vi "SetNeoPixelBrightness.vi"(8 "error in (no error)":errorcluster, 10 "Brightness":u8, 11 "AdaFruit-Seesaw in":refnum<class "AdaFruit-Seesaw.lvclass">) -> (0 "error out":errorcluster, 3 "AdaFruit-Seesaw out":refnum<class "AdaFruit-Seesaw.lvclass">)   [LabVIEW 2020, in "CTI-Peripheral.lvlib" / "AdaFruit-Seesaw.lvclass"]
uses:
  AdaFruit-Seesaw.lvclass
  AdaFruit-Seesaw.lvclass/AdaFruit-Seesaw.ctl
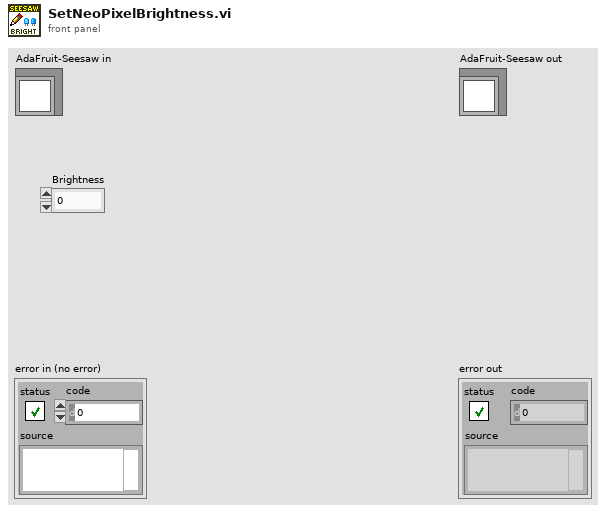
[diagram p1: front panel]
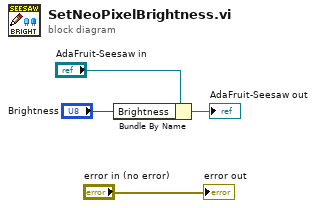
[diagram p0: block diagram]
diagram:
  n1 = Bundle By Name(cluster="AdaFruit-Seesaw in", "Brightness"="Brightness") -> (→"AdaFruit-Seesaw out":refnum<class "AdaFruit-Seesaw.lvclass">)
  "error out" <- "error in (no error)"
